vi "Write Pulse Configuration.vi"(8 "error in (no error)":errorcluster, 10 "Configuration":T1={"Pre-trigger duration"=0.01, "Post-trigger duration"=0.1, "Rate"=1000000.0, "Ranges"=[10.0], "Re-name channels"=[], "Active channels"="0:1", "External clock"=FALSE} {"Rate" format="%#_8pHz"; "Post-trigger duration" format="%#_6ps"; "Pre-trigger duration" format="%#_6ps"; "Ranges" format="%#_6pV"}, 11 "Red Pitaya Modulated Digitizer in":refnum<class "Red Pitaya Modulated Digitizer.lvclass">) -> (0 "error out":errorcluster, 3 "Red Pitaya Modulated Digitizer out":refnum<class "Red Pitaya Modulated Digitizer.lvclass">)   [LabVIEW 2020, in "Red Pitaya Modulated Digitizer.lvclass"]
uses:
  Red Pitaya Modulated Digitizer.lvclass
  Instruments/Pulse Driver/Pusle Driver Configuration.ctl
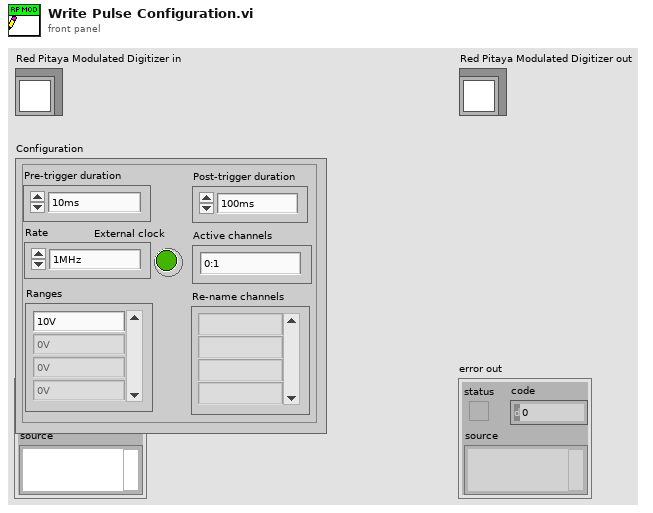
[diagram p1: front panel]
types:
  T1 = typedef "Pusle Driver Configuration.ctl" = cluster{"Pre-trigger duration":dbl, "Post-trigger duration":dbl, "Rate":dbl, "Ranges":dbl[], "Re-name channels":string[], "Active channels":string, "External clock":bool}
  T2 = typedef "RP Modulated Configuration.ctl" = cluster{"Pre-trigger duration":dbl, "Post-trigger duration":dbl, "Rate":dbl, "Ranges":dbl[], "Re-name channels":string[], "Active channels":string, "External clock":bool, "Modulation":T3}
  T3 = typedef "Modulation.ctl" = cluster{"Output delay":dbl, "After delay":bool}
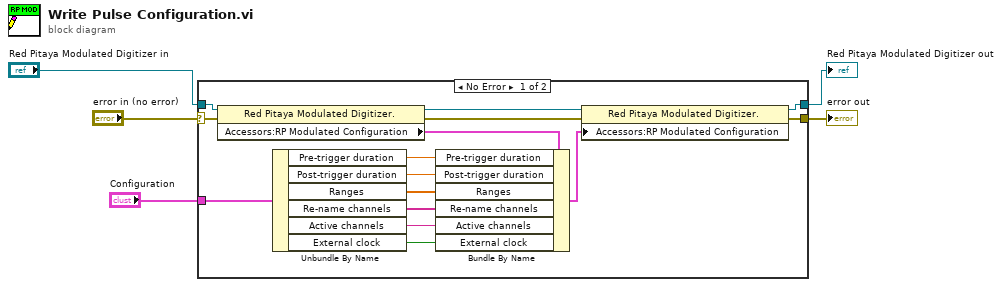
[diagram p0: block diagram]
diagram:
  n1 = case shown="No Error" "error in (no error)" {
    selector: "error in (no error)" -> [w9 w21]
    tunnel: [w8 w21] -> w4
    tunnel: [w7 w22] -> w2
    tunnel: "Red Pitaya Modulated Digitizer in" -> [w6 w22]
    tunnel: "Configuration" -> [w18 _]
    frame No Error {
      n2 = property class="Red Pitaya Modulated Digitizer."(reference=w6, error in=w9) -> (reference out=w20:refnum<class "Red Pitaya Modulated Digitizer.lvclass">, error out=w19:errorcluster, "Accessors:RP Modulated Configuration"=w14:T2)
      n3 = Unbundle By Name(w18) -> ("Pre-trigger duration"=w17:dbl, "Post-trigger duration"=w16:dbl, "Ranges"=w15:dbl[], "Re-name channels"=w13:string[], "Active channels"=w12:string, "External clock"=w11:bool)
      n4 = Bundle By Name(cluster=w14, "Pre-trigger duration"=w17, "Post-trigger duration"=w16, "Ranges"=w15, "Re-name channels"=w13, "Active channels"=w12, "External clock"=w11) -> (w10:T2)
      n5 = property class="Red Pitaya Modulated Digitizer."(reference=w20, error in=w19, "Accessors:RP Modulated Configuration"=w10) -> (reference out=w7:refnum<class "Red Pitaya Modulated Digitizer.lvclass">, error out=w8:errorcluster)
    }
    frame Error {
    }
  }
  "error out" <- w4
  "Red Pitaya Modulated Digitizer out" <- w2
